vi "encodeArray.vi"(6 "MsgPack Config":T1={"Cluster Conversion"=enum."to array", "Enum Conversion"=enum."to uint", "Use ArrayType"=FALSE}, 8 "error in (no error)":errorcluster, 10 "Variant":variant) -> (0 "error out":errorcluster, 2 "Array":u8[](array[numeric]) format="%.0x")   [LabVIEW 2016, in "MsgPack.lvlib"]
uses:
  MsgPack.lvlib
  SubVis/msgpack_config.ctl
  SubVis/cluster_conversion.ctl
  SubVis/enum_conversion.ctl
  <userlib>/_OpenG.lib/lvdata/lvdata.llb/Type Descriptor Enumeration__ogtk.ctl
  <vilib>/Utility/error.llb/Error Cluster From Error Code.vi
  enc_a_I8.vi
  enc_a_I16.vi
  enc_a_I32.vi
  enc_a_I64.vi
  enc_a_U8.vi
  enc_a_U16.vi
  enc_a_U32.vi
  enc_a_U64.vi
  enc_a_FloatSgl.vi
  <vilib>/ErrorRing/Error Ring.xnode
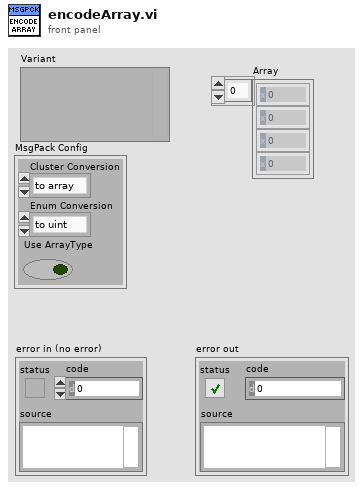
[diagram p1: front panel]
types:
  T1 = typedef "MsgPack.lvlib/msgpack_config.ctl" = cluster{"Cluster Conversion":T2, "Enum Conversion":T3, "Use ArrayType":bool}
  T2 = typedef "MsgPack.lvlib/cluster_conversion.ctl" = enum16{"to map", "to array"}
  T3 = typedef "MsgPack.lvlib/enum_conversion.ctl" = enum16{"to uint", "to string"}
  T4 = typedef "Type Descriptor Enumeration__ogtk.ctl" = enum8{"<Null>", "I8", "I16", "I32", "I64", "U8", "U16", "U32", "U64", "SGL", "DBL", "EXT", "CSG", "CDB", "CXT", "0x0F", "0x10", "0x11", "0x12", "0x13", "0x14", "Enum U8", "Enum U16", "Enum U32", "Enum U64", "SGL PQ", "DBL PQ", "EXT PQ", "CSG PQ", "CDB PQ", "CXT PQ", "0x1F", "0x20", "Boolean", "0x22", "0x23", "0x24", "0x25", "0x26", "0x27", "0x28", "0x29", "0x2A", "0x2B", "0x2C", "0x2D", "0x2E", "0x2F", "String", "0x31", "Path", "Pict", "0x34", "0x35", "0x36", "DAQ", "0x38", "0x39", "0x3A", "0x3B", "0x3C", "0x3D", "0x3E", "0x3F", "Array", "0x41", "0x42", "0x43", "0x44", "0x45", "0x46", "0x47", "0x48", "0x49", "0x4A", "0x4B", "0x4C", "0x4D", "0x4E", "0x4F", "Cluster", "0x51", "0x52", "Variant", "Waveform", "0x55", "0x56", "0x57", "0x58", "0x59", "0x5A", "0x5B", "0x5C", "0x5D", "0x5E", "0x5F", "0x60", "0x61", "0x62", "0x63", "0x64", "0x65", "0x66", "0x67", "0x68", "0x69", "0x6A", "0x6B", "0x6C", "0x6D", "0x6E", "0x6F", "Refnum"}
  T5 = typedef "Type Descriptor__ogtk.ctl" = i16[]
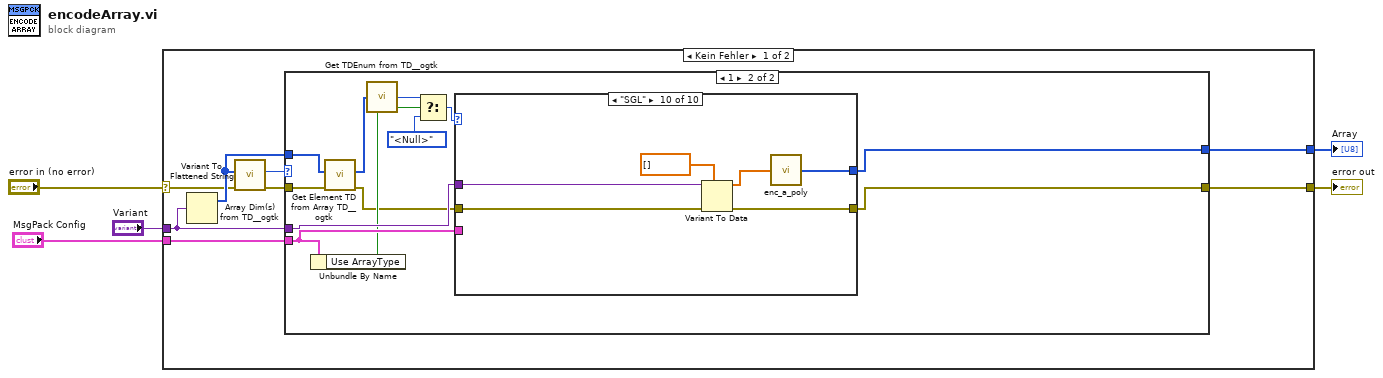
[diagram p0: block diagram]
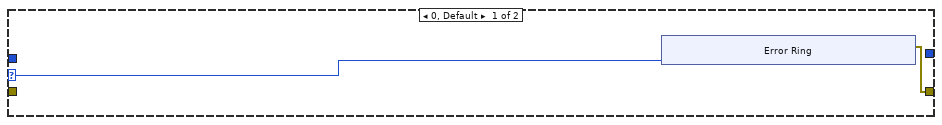
[diagram p2: hidden frame]
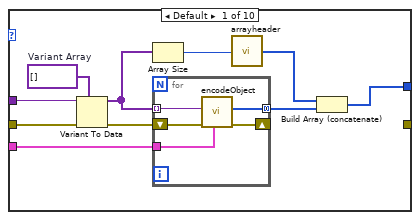
[diagram p3: hidden frame]
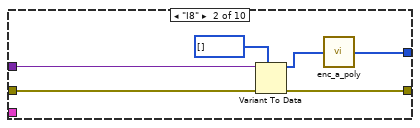
[diagram p4: hidden frame]
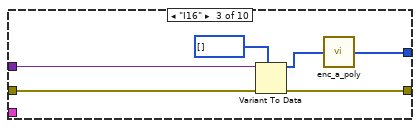
[diagram p5: hidden frame]
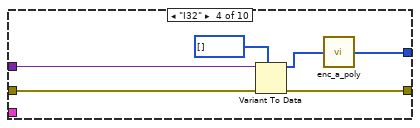
[diagram p6: hidden frame]
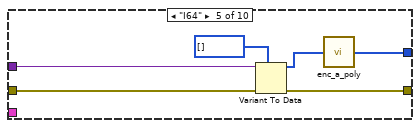
[diagram p7: hidden frame]
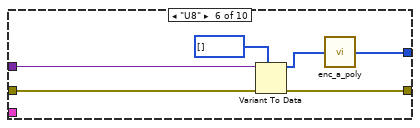
[diagram p8: hidden frame]
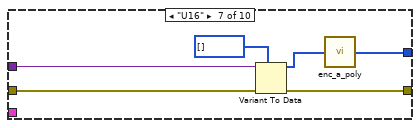
[diagram p9: hidden frame]
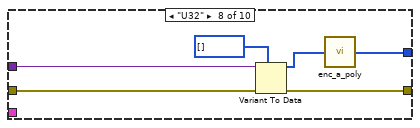
[diagram p10: hidden frame]
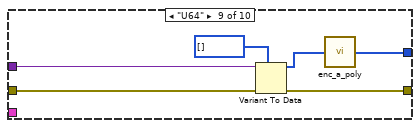
[diagram p11: hidden frame]
diagram:
  n1 = case shown="Kein Fehler" "error in (no error)" {
    selector: "error in (no error)" -> [w6 w104]
    tunnel: [w9 _] -> w5
    tunnel: [w13 w104] -> w4
    tunnel: "Variant" -> [w8 _]
    tunnel: "MsgPack Config" -> [w12 _]
    frame No Error {
      n2 = Variant To Flattened String(Variant=w8) -> (1:w7:i16[])  [unwired: 1 out]
      n3 = call <userlib>:"Array Dim(s) from TD__ogtk.vi"("error in (no error)"=w6, "Array Type Descriptor"=w7) -> ("error out"=w10:errorcluster, "N dims"=w11:u32)  [unwired: 8 in]
      n4 = case shown="1" w11 {
        selector: w11 -> [w14 _]
        tunnel: w10 -> [_ w24]
        tunnel: [w15 w33] -> w13
        tunnel: w8 -> [_ w34]
        tunnel: [_ w32] -> w9
        tunnel: w12 -> [_ w28]
        tunnel: w7 -> [_ w25]
        frame 0, Default {
          n5 = xnode "Error Ring"("Parameter 0"=w14) -> ("Fehler (Ausgang)"=w15:errorcluster)
        }
        frame 1 {
          n6 = Unbundle By Name(w28) -> ("Use ArrayType"=w27:bool)
          n7 = call <userlib>:"Get Element TD from Array TD__ogtk.vi"("error in (no error)"=w24, "Array Type Descriptor"=w25) -> ("error out"=w23:errorcluster, "Element Type Descriptor"=w26:T5)  [unwired: 8 in]
          n8 = call <userlib>:"Get TDEnum from TD__ogtk.vi"("Type Descriptor"=w26) -> ("Type Descriptor Enumeration"=w31:T4)  [unwired: 4 in]
          n9 = Select(t=w31, s=w27, f=Type_Descriptor_Enumeration__ogtk."<Null>") -> (s? t:f=w30:T4)
          n10 = case shown="\"SGL\"" w30 {
            tunnel: w34 -> [w38 w55 w61 w67 w73 w79 w85 w91 w97 w103]
            tunnel: [w36 w51 w57 w63 w69 w75 w81 w87 w93 w99] -> w32
            tunnel: [_ w52 w59 w64 w70 w76 w82 w88 w94 w100] -> w33
            tunnel: w28 -> [w37 _ _ _ _ _ _ _ _ _]
            tunnel: w23 -> [w35 w50 w56 w62 w68 w74 w80 w86 w92 w98]
            frame Default {
              w39 = variant[] []  # Variant Array
              n11 = Variant To Data(error in=w35, type=w39, Variant=w38) -> (data=w41:variant[], error out=w40:errorcluster)
              n12 = Array Size(array=w41) -> (size(s)=w42:i32)
              n13 = for {
                shift-right: [w49] -> _
                shift-left: w40 -> [w46]
                tunnel: [w48] -> w43 mode=concatenating
                tunnel: w37 -> [w47]
                tunnel: w41 -> [w45] mode=indexing
                n14 = call "encodeObject.vi"("MsgPack Config"=w47, "error in (no error)"=w46, "Variant"=w45) -> ("error out"=w49:errorcluster, "Array"=w48:u8[])  [unwired: 7 in]
              }
              n15 = call "arrayheader.vi"("Number of Elements"=w42) -> ("header"=w44:u8[])
              n16 = Build Array (concatenate)(w44, w43) -> (w36:u8[])
            }
            frame "I8" {
              n17 = Variant To Data(error in=w50, type=i8[] [], Variant=w55) -> (data=w53:i8[], error out=w52:errorcluster)
              n18 = call-poly "enc_a_poly.vi"("Array In"=w53) -> ("Array Out"=w51:u8[])
            }
            frame "I16" {
              n19 = Variant To Data(error in=w56, type=i16[] [], Variant=w61) -> (data=w58:i16[], error out=w59:errorcluster)
              n20 = call-poly "enc_a_poly.vi"("Array In"=w58) -> ("Array Out"=w57:u8[])
            }
            frame "I32" {
              n21 = Variant To Data(error in=w62, type=i32[] [], Variant=w67) -> (data=w65:i32[], error out=w64:errorcluster)
              n22 = call-poly "enc_a_poly.vi"("Array In"=w65) -> ("Array"=w63:u8[])
            }
            frame "I64" {
              n23 = Variant To Data(error in=w68, type=i64[] [], Variant=w73) -> (data=w71:i64[], error out=w70:errorcluster)
              n24 = call-poly "enc_a_poly.vi"("Array In"=w71) -> ("Array Out"=w69:u8[])
            }
            frame "U8" {
              n25 = Variant To Data(error in=w74, type=u8[] [], Variant=w79) -> (data=w77:u8[], error out=w76:errorcluster)
              n26 = call-poly "enc_a_poly.vi"("Array In"=w77) -> ("Array Out"=w75:u8[])
            }
            frame "U16" {
              n27 = Variant To Data(error in=w80, type=u16[] [], Variant=w85) -> (data=w83:u16[], error out=w82:errorcluster)
              n28 = call-poly "enc_a_poly.vi"("Array In"=w83) -> ("Array Out"=w81:u8[])
            }
            frame "U32" {
              n29 = Variant To Data(error in=w86, type=u32[] [], Variant=w91) -> (data=w89:u32[], error out=w88:errorcluster)
              n30 = call-poly "enc_a_poly.vi"("Array In"=w89) -> ("Array Out"=w87:u8[])
            }
            frame "U64" {
              n31 = Variant To Data(error in=w92, type=u64[] [], Variant=w97) -> (data=w95:u64[], error out=w94:errorcluster)
              n32 = call-poly "enc_a_poly.vi"("Array In"=w95) -> ("Array Out"=w93:u8[])
            }
            frame "SGL" {
              n33 = Variant To Data(error in=w98, type=sgl[] [], Variant=w103) -> (data=w101:sgl[], error out=w100:errorcluster)
              n34 = call-poly "enc_a_poly.vi"("Array In"=w101) -> ("Array Out"=w99:u8[])
            }
          }
        }
      }
    }
    frame Error {
    }
  }
  "Array" <- w5
  "error out" <- w4
